vi "WebFrontPanel_Create.vi"(0 "reference in":refnum<class "WebFrontPanel.lvclass">, 1 "VI Name":string, 5 "error in (no error)":errorcluster, 8 "VI Reference":refnum<vi>) -> (14 "reference out":refnum<class "WebFrontPanel.lvclass">, 19 "error out":errorcluster)   [LabVIEW 2014, in "WebFrontPanel.lvclass"]
uses:
  WebFrontPanel.lvclass
  Object_class/Object.lvclass
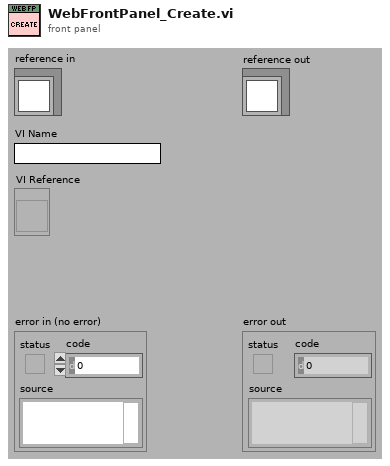
[diagram p1: front panel]
types:
  T1 = typedef "WebFrontPanel.lvclass/ObjectAttributes.ctl" = cluster{"VI Name":string, "VI Reference":refnum<vi>, "Controls":refnum<class "Object.lvclass">[], "Indicators":refnum<class "Object.lvclass">[], "Decorations":refnum<class "Object.lvclass">[]}
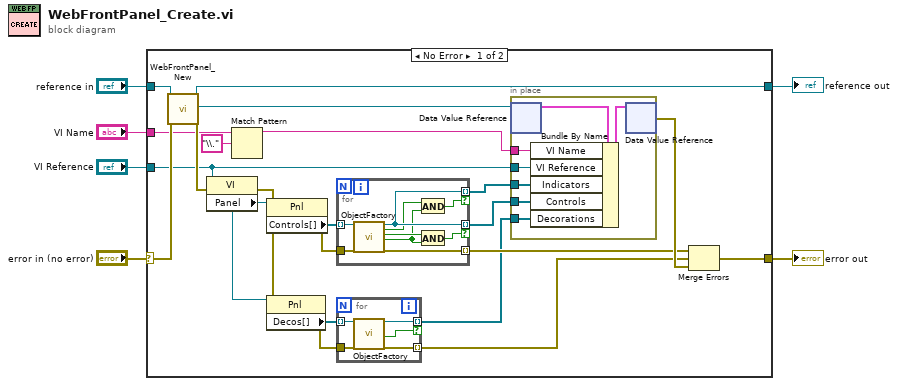
[diagram p0: block diagram]
diagram:
  n1 = case shown="No Error" "error in (no error)" {
    selector: "error in (no error)" -> [w28 w51]
    tunnel: [w26 w51] -> w5
    tunnel: "reference in" -> [w21 w50]
    tunnel: [w20 w50] -> w3
    tunnel: "VI Name" -> [w8 _]
    tunnel: "VI Reference" -> [w18 _]
    frame No Error {
      n2 = call "WebFrontPanel_New.vi"("reference in"=w21, "error in (no error)"=w28) -> ("reference out"=w20:refnum<class "WebFrontPanel.lvclass">, "DVRRefOut"=w19:refnum<data-value>, "error out"=w25:errorcluster)  [unwired: 14 in, 1 out]
      n3 = property class="VI"(reference=w18, error in=w25) -> (error out=w23:errorcluster, "Panel"=w16:refnum<vi>)  [unwired: 1 out]
      n4 = Match Pattern(string=w8, regular expression="\\.") -> (before substring=w7:string)  [unwired: 1 in, 3 out]
      n5 = property class="Pnl"(reference=w16, error in=w23) -> (error out=w24:errorcluster, "Controls[]"=w17:refnum<vi>[])  [unwired: 1 out]
      n6 = property class="Pnl"(reference=w16, error in=w23) -> (error out=w22:errorcluster, "Decos[]"=w15:refnum<vi>[])  [unwired: 1 out]
      n7 = for {
        tunnel: w17 -> [w39] mode=indexing
        tunnel: [w40] -> w12 mode=indexing if=w37
        tunnel: [w40] -> w11 mode=indexing if=w34
        tunnel: w24 -> [w42]
        tunnel: [w41] -> w14 mode=indexing
        n8 = call "ObjectFactory.vi"("GOject"=w39, "error in (no error)"=w42) -> ("Object"=w40:refnum<class "Object.lvclass">, "Is Indicator"=w38:bool, "Is Control"=w36:bool, "Is Visible"=w35:bool, "error out"=w41:errorcluster)  [unwired: 13 in]
        n9 = And(x=w38, y=w35) -> (x .and. y?=w37:bool)
        n10 = And(x=w36, y=w35) -> (x .and. y?=w34:bool)
      }
      n11 = for {
        tunnel: w15 -> [w31] mode=indexing
        tunnel: [w30] -> w10 mode=indexing if=w29
        tunnel: w22 -> [w33]
        tunnel: [w32] -> w13 mode=indexing
        n12 = call "ObjectFactory.vi"("GOject"=w31, "error in (no error)"=w33) -> ("Object"=w30:refnum<class "Object.lvclass">, "Is Visible"=w29:bool, "error out"=w32:errorcluster)  [unwired: 13 in, 2 out]
      }
      n13 = in-place {
        in-place-border: w7 -> [w47]
        in-place-border: w18 -> [w46]
        in-place-border: w12 -> [w45]
        in-place-border: w11 -> [w44]
        in-place-border: w10 -> [w43]
        n14 = in-place-dvr #1(w19) -> (w48:T1)  [unwired: 1 out]
        n15 = Bundle By Name(cluster=w48, "VI Name"=w47, "VI Reference"=w46, "Indicators"=w45, "Controls"=w44, "Decorations"=w43) -> (w49:T1)
        n16 = in-place-dvr #1(w49) -> (w27:errorcluster)  [unwired: 1 out]
      }
      n17 = Merge Errors(w14, w13, w27) -> (w26:errorcluster)
    }
    frame Error {
    }
  }
  "error out" <- w5
  "reference out" <- w3
